vi "TxtFile Append.vi"(8 "error in (no error)":errorcluster, 10 "Content":string, 11 "Config File dir":path) -> (0 "error out":errorcluster, 3 "config file path":path)   [LabVIEW 2012]
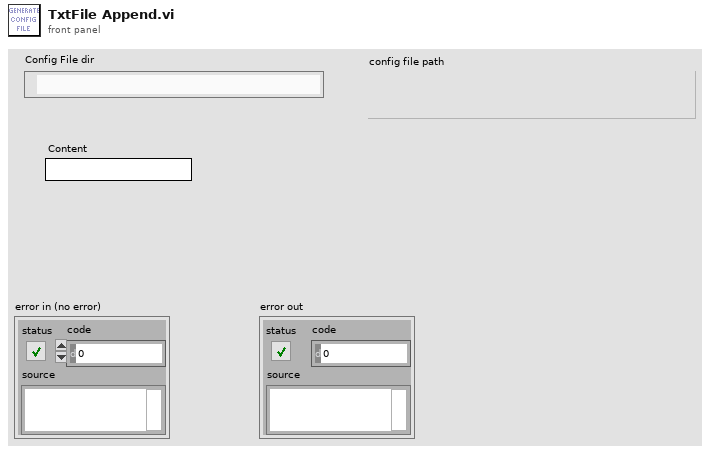
[diagram p1: front panel]
types:
  T1 = enum16{"open", "replace", "create", "open or create", "replace or create", "replace or create with confirmation"}
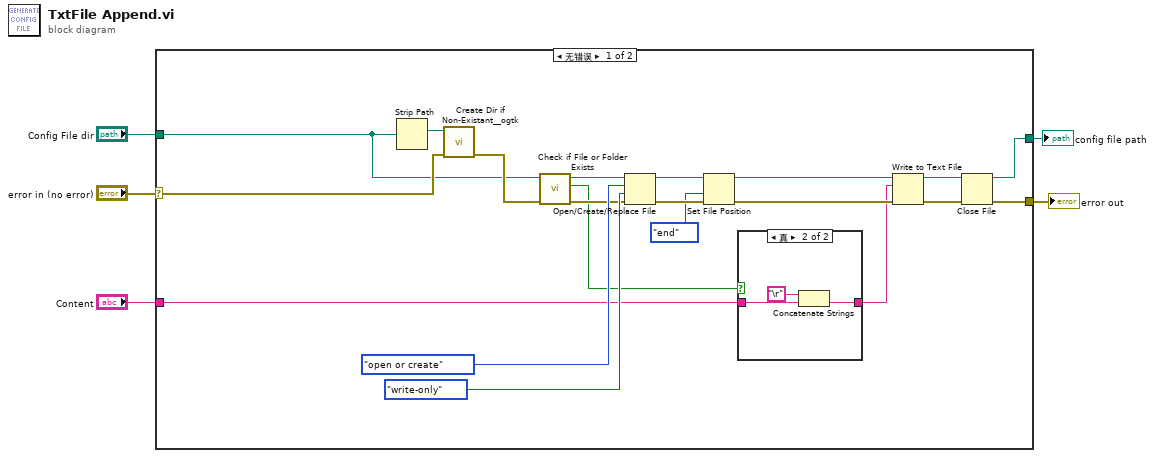
[diagram p0: block diagram]
diagram:
  n1 = case shown="无错误" "error in (no error)" {
    selector: "error in (no error)" -> [w8 w30]
    tunnel: [w21 w30] -> w4
    tunnel: [w13 _] -> w3
    tunnel: "Config File dir" -> [w7 _]
    tunnel: "Content" -> [w6 _]
    frame No Error {
      n2 = Strip Path(path=w7) -> (stripped path=w14:path)  [unwired: 1 out]
      n3 = call <userlib>:"Create Dir if Non-Existant__ogtk.vi"("error in (no error)"=w8, "Directory Path"=w14) -> ("error out"=w11:errorcluster)  [unwired: 7 in, 2 out]
      n4 = call <vilib>:"Check if File or Folder Exists.vi"("error in (no error)"=w11, "path"=w7) -> ("error out"=w10:errorcluster, "file or folder exists?"=w9:bool, "dup path"=w12:path)  [unwired: 7 in]
      n5 = Open/Create/Replace File(file path (use dialog)=w12, error in=w10, operation (0:open)=T1."open or create", access (0:read/write)=enum16{"read/write", "read-only", "write-only"}."write-only") -> (refnum out=w16:refnum<file>, error out=w18:errorcluster)  [unwired: 2 in, 1 out]
      n6 = Set File Position(refnum=w16, from (0:start)=enum16{"start", "end", "current"}."end", error in=w18) -> (refnum out=w20:refnum<file>, error out=w19:errorcluster)  [unwired: 1 in]
      n7 = case shown="真" w9 {
        tunnel: w6 -> [w26 w28]
        tunnel: [w26 w27] -> w15
        frame False {
        }
        frame True {
          n8 = Concatenate Strings("\r" ("Carriage Return Constant"), w28) -> (w27:string)
        }
      }
      n9 = Write to Text File(file (use dialog)=w20, text=w15, error in=w19) -> (refnum out=w23:refnum<file>, error out=w22:errorcluster)  [unwired: 1 in, 1 out]
      n10 = Close File(refnum=w23, error in=w22) -> (path=w13:path, error out=w21:errorcluster)
    }
    frame Error {
    }
  }
  "error out" <- w4
  "config file path" <- w3
